vi "Set Home Impl.vi"(8 "error in (no error)":errorcluster, 11 "ASI Stage in":refnum<class "ASI Stage.lvclass">) -> (0 "error out":errorcluster, 3 "ASI Stage out":refnum<class "ASI Stage.lvclass">)   [LabVIEW 2023, in "ASI Stage.lvlib" / "ASI Stage.lvclass"]
uses:
  ASI Stage.lvclass
  ASI Stage.lvclass/ASI Stage.ctl
  <instrlib>/ASI TG-1000/ASI TG-1000.lvlib
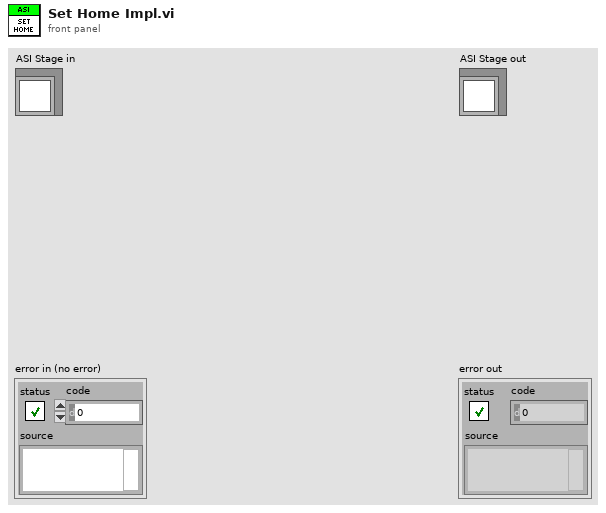
[diagram p1: front panel]
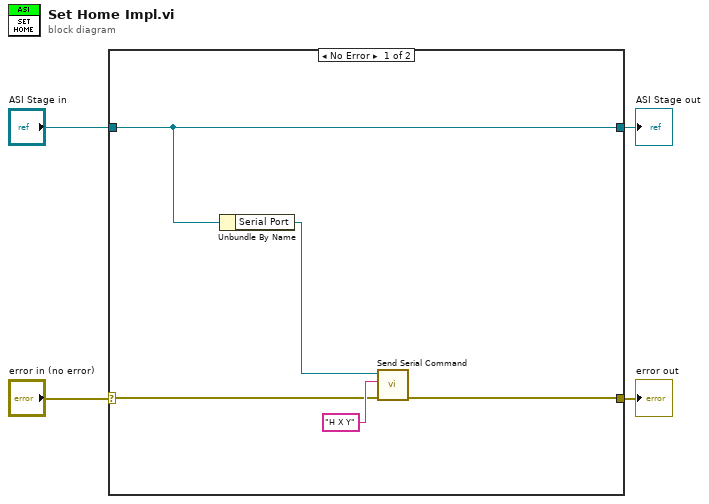
[diagram p0: block diagram]
diagram:
  n1 = case shown="No Error" "error in (no error)" {
    selector: "error in (no error)" -> [w8 w11]
    tunnel: "ASI Stage in" -> [w6 w10]
    tunnel: [w6 w10] -> w3
    tunnel: [w7 w11] -> w1
    frame No Error {
      n2 = Unbundle By Name(w6) -> ("Serial Port"=w5:refnum<visa-resource-name>)
      n3 = call <instrlib>:"Send Serial Command.vi"("error in (no error)"=w8, "Command"="H X Y", "VISA in"=w5) -> ("error out"=w7:errorcluster)  [unwired: 6 in, 2 out]
    }
    frame Error {
    }
  }
  "error out" <- w1
  "ASI Stage out" <- w3
